vi "Build_Request.vi"(8 "error in (no error)":errorcluster, 11 "Asana in":refnum<class "Asana.lvclass">) -> (0 "error out":errorcluster, 3 "Asana out":refnum<class "Asana.lvclass">)   [LabVIEW 2016, in "Asana.lvclass"]
uses:
  Asana.lvclass
  Asana.lvclass/Asana.ctl
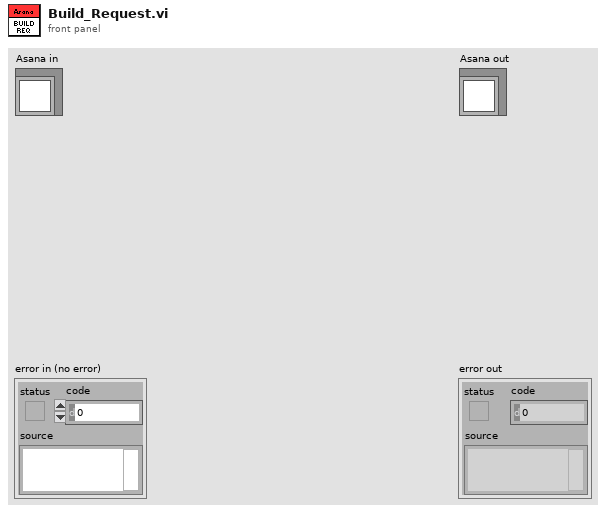
[diagram p1: front panel]
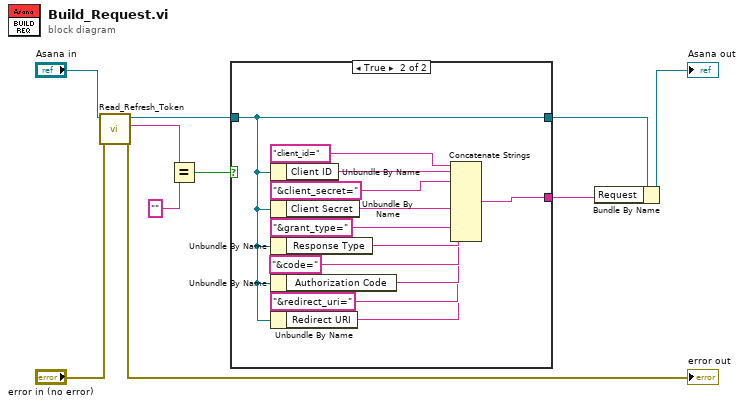
[diagram p0: block diagram]
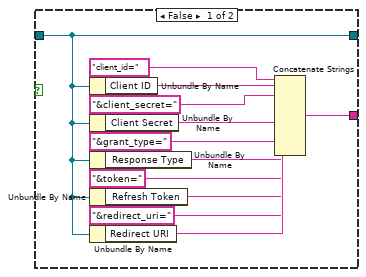
[diagram p2: hidden frame]
diagram:
  n1 = call-dynamic "Read_Refresh_Token.vi"("error in (no error)"="error in (no error)", "Asana in"="Asana in") -> ("error out"=→"error out":errorcluster, "Refresh Token"=w7:string, "Asana out"=w1:refnum<class "Asana.lvclass">)  [unwired: 7 in]
  n2 = Equal?(x=w7, y="") -> (x = y?=w5:bool)
  n3 = case shown="True" w5 {
    tunnel: [w11 w26] -> w3
    tunnel: [w12 w23] -> w4
    tunnel: w1 -> [w11 w26]
    frame False {
      n4 = Unbundle By Name(w11) -> ("Client ID"=w14:string)
      n5 = Unbundle By Name(w11) -> ("Client Secret"=w16:string)
      n6 = Unbundle By Name(w11) -> ("Response Type"=w18:string)
      n7 = Unbundle By Name(w11) -> ("Refresh Token"=w20:string)
      n8 = Unbundle By Name(w11) -> ("Redirect URI"=w22:string)
      n9 = Concatenate Strings("client_id=", w14, "&client_secret=" ("string"), w16, "&grant_type=" ("string"), w18, "&token=" ("string"), w20, "&redirect_uri=" ("string"), w22) -> (w12:string)
    }
    frame True {
      n10 = Unbundle By Name(w26) -> ("Client ID"=w33:string)
      n11 = Unbundle By Name(w26) -> ("Client Secret"=w31:string)
      n12 = Unbundle By Name(w26) -> ("Response Type"=w29:string)
      n13 = Unbundle By Name(w26) -> ("Authorization Code"=w27:string)
      n14 = Unbundle By Name(w26) -> ("Redirect URI"=w24:string)
      n15 = Concatenate Strings("client_id=", w33, "&client_secret=" ("string"), w31, "&grant_type=" ("string"), w29, "&code=" ("string"), w27, "&redirect_uri=" ("string"), w24) -> (w23:string)
    }
  }
  n16 = Bundle By Name(cluster=w3, "Request"=w4) -> (→"Asana out":refnum<class "Asana.lvclass">)
